vi "Actor Core.vi"(8 "error in":errorcluster, 11 "Example Actor in":refnum<class "Example Actor.lvclass">) -> (0 "error out":errorcluster, 3 "Actor out":refnum<class "Actor.lvclass">)   [LabVIEW 2021, in "Example Iterator NR Actor Explicit Iteration.lvlib" / "Example Actor.lvclass"]
doc: "(<B>Filename</B>: Actor Framework.lvlib:Actor.lvclass:Actor Core.vi)\n\nReceives messages to the actor, reacts to them, and initiates any error handling that may shut the actor down.\n\nDescendant classes may override this VI to append parallel tasks for the actor to complete while it handles messages. Overrides use the Call Parent Method node."
uses:
  Example Actor.lvclass
  C:/Program Files/National Instruments/LabVIEW 2021/vi.lib/ActorFramework/Actor/Actor.lvclass
  <vilib>/ActorFramework/Actor/Actor.lvclass
  Iterator Settings.ctl
  Abstract Iterator Actor/Active Stop Conditions.ctl
  Abstract Iterator Actor/Stop Reason.ctl
  Iterator NR Actor/Iterator NR Actor Folder/Iterator NR Actor.lvclass
  Example Actor.lvclass/Example Actor.ctl
  <vilib>/ActorFramework/Actor/Actor.lvclass/Actor.ctl
  <vilib>/ActorFramework/Message Enqueuer/Message Enqueuer.lvclass/Message Enqueuer.ctl
  Example Actor Messages/Iterate Reply Msg/Iteration Msg.lvclass
  C:/Program Files/National Instruments/LabVIEW 2021/vi.lib/ActorFramework/Message/Message.lvclass
  Abstract Iterator Actor/Iterator Settings.ctl
  <vilib>/ActorFramework/Message/Message.lvclass
  Iterator Actor/Iterator Actor Abstract Messages/Iterator Report Iterations End Msg/Iterator Report Iterations End Msg.lvclass
  Example Actor Messages/Pre Iterate Reply Msg/Pre Iteration Msg.lvclass
  Example Actor Messages/Post Iterate Reply Msg/Post Iteration Msg.lvclass
  Example Actor Messages/Update Error Msg/Update Error Msg.lvclass
  C:/Projects/Shared Libraries/Iterator Actor/Iterator Actor/Iterator Actor Abstract Messages/Iterator Report Iterations End Msg/Iterator Report Iterations End Msg.lvclass
  <vilib>/ActorFramework/Message Enqueuer/Init from Existing Queue.vi
  <vilib>/ActorFramework/Message Enqueuer/Enqueue.vi
  <vilib>/ActorFramework/Stop Msg/Stop Msg.lvclass
  <vilib>/ActorFramework/Message Priority Queue/Priority Enqueue.vi
  <vilib>/ActorFramework/Message Enqueuer/Message Enqueuer.lvclass
  Example Actor Messages/Write Ready for iterations Msg/Write Ready for iterations Msg.lvclass
  Iterator Actor/Iterator Actor Messages/Write Settings Msg/Write Settings Msg.lvclass
  Iterator Actor/Iterator Actor Messages/Start Iterations Msg/Start Iterations Msg.lvclass
  Iterator Actor/Iterator Actor Messages/Stop Iterations Msg/Stop Iterations Msg.lvclass
  Abstract Iterator Actor/Abstract Iterator Actor.lvclass
panel:
  out "Stop Reason":T1
  in  "Receive report":bool=TRUE
  in  "Do post-iterations":bool=TRUE
  in  "Do pre-iterations":bool=TRUE
  out "Iterator error":errorcluster
  in  "User Settings":T2={"Prepare timeout (ms)"=1000, "Iterate timeout (ms)"=1000, "Conclude timeout (ms)"=1000, "Iterate period (ms)"=1000, "Active Stop Conditions"={"Number of Iterations"=FALSE, "Time Elapsed"=FALSE, "Iteration Result"=FALSE}, "Iterations"=5, "Time before stop (ms)"=200}
  out "Post Iterate":bool
  out "Pre Iterate":bool
  in  "exit":bool
  out "Iterate":bool
  in  "stop iterations":bool
  in  "start iterations":bool
  in  "Ready for iterations":bool=TRUE
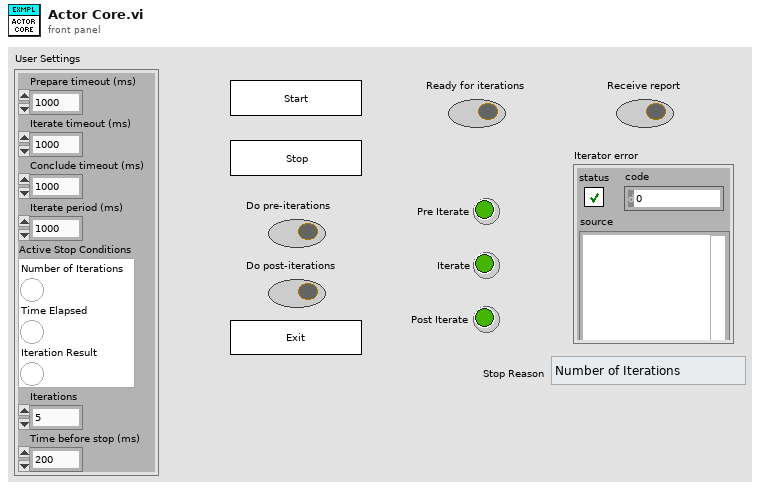
[diagram p1: front panel]
types:
  T1 = typedef "Iterator Actor.lvlib/Abstract Iterator Actor.lvclass/Stop Reason.ctl" = enum16{"Number of Iterations", "Time Elapsed", "Stopped Internally", "Stopped Externally"}
  T2 = typedef "Example Iterator NR Actor Explicit Iteration.lvlib/Example Actor.lvclass/Iterator Settings.ctl" = cluster{"Prepare timeout (ms)":i32, "Iterate timeout (ms)":i32, "Conclude timeout (ms)":i32, "Iterate period (ms)":i32, "Active Stop Conditions":T3, "Iterations":i32, "Time before stop (ms)":i32}
  T3 = typedef "Iterator Actor.lvlib/Abstract Iterator Actor.lvclass/Active Stop Conditions.ctl" = cluster{"Number of Iterations":bool, "Time Elapsed":bool, "Iteration Result":bool}
  T4 = typedef "Iterator Actor.lvlib/Abstract Iterator Actor.lvclass/Iterator Settings.ctl" = cluster{"Prepare timeout (ms)":i32, "Iterate timeout (ms)":i32, "Conclude timeout (ms)":i32, "Iterate period (ms)":i32, "Number of iterations":i32, "Time before stop (ms)":i32, "Active Stop Conditions":T3, "Prepare Msg":refnum<class "Message.lvclass">, "Iterate Msg":refnum<class "Message.lvclass">, "Conclude Msg":refnum<class "Message.lvclass">, "Iterations End Report":refnum<class "Iterator Report Iterations End Msg.lvclass">}
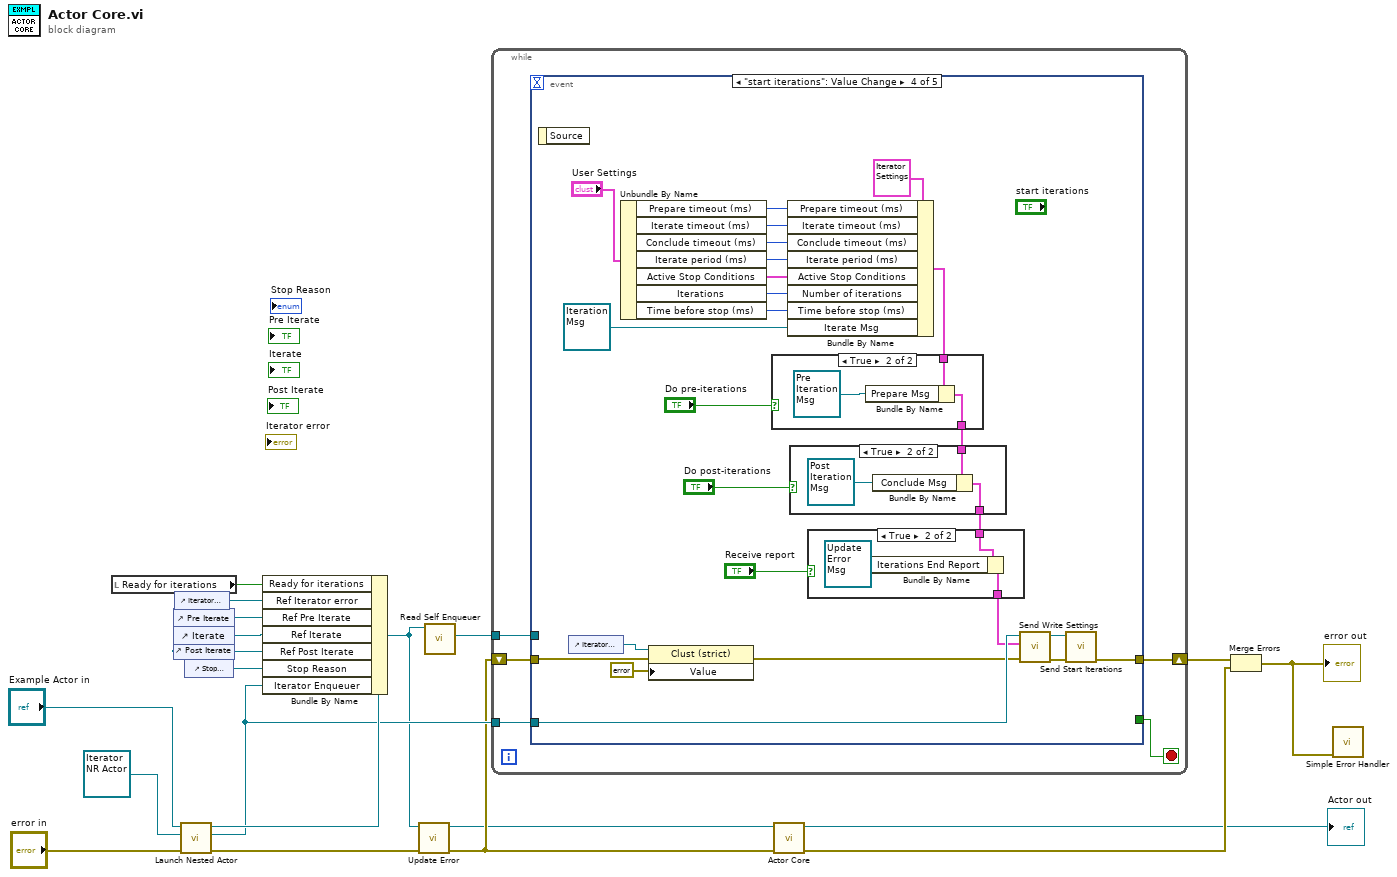
[diagram p0: block diagram]
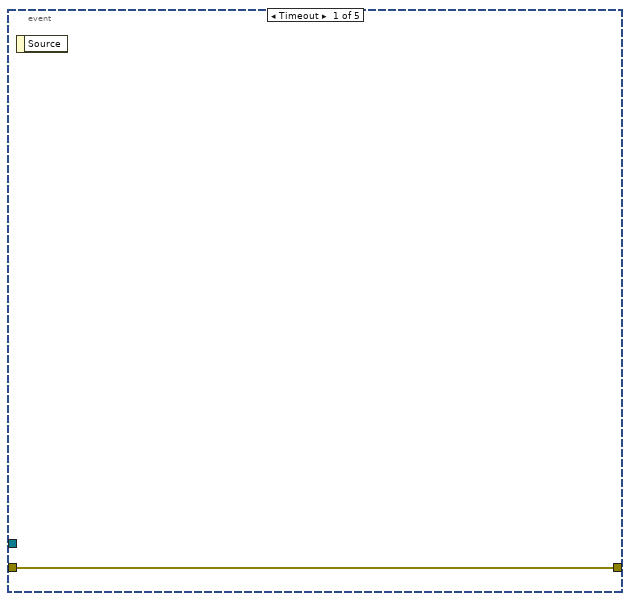
[diagram p2: hidden frame]
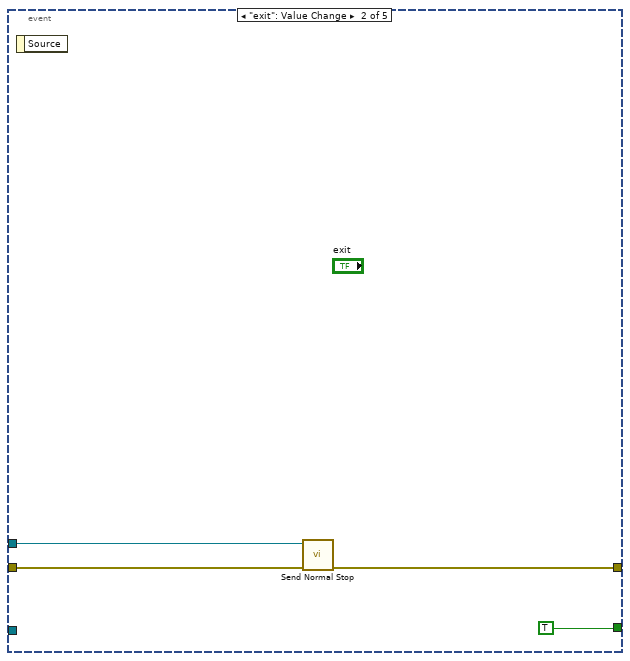
[diagram p3: hidden frame]
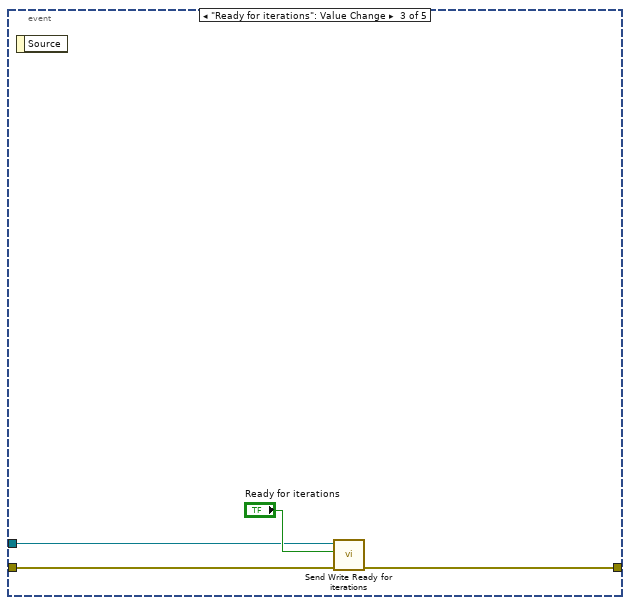
[diagram p4: hidden frame]
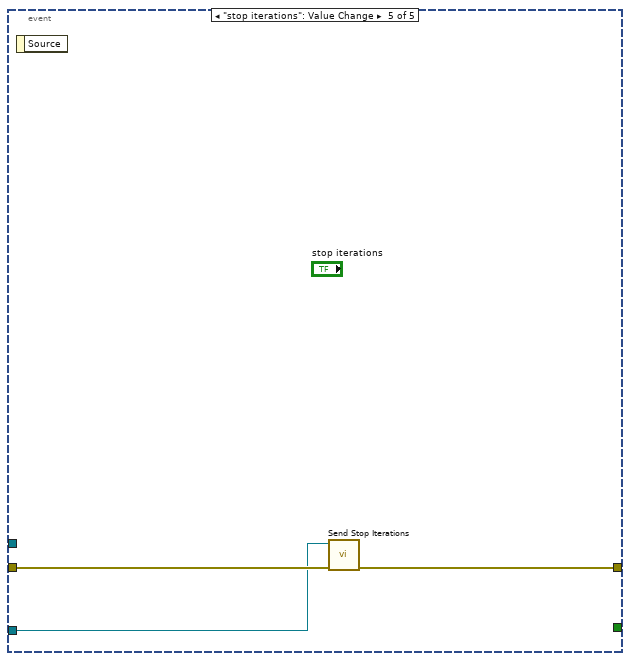
[diagram p8: hidden frame]
diagram:
  n1 = local read "Ready for iterations"() -> (w11:bool)
  n2 = control-ref of="Pre Iterate"() -> (w16:refnum<vi>)
  n3 = control-ref of="Iterate"() -> (w15:refnum<vi>)
  n4 = control-ref of="Post Iterate"() -> (w14:refnum<vi>)
  n5 = control-ref of="Iterator error"() -> (w9:refnum<vi>)
  n6 = call <vilib>:"Launch Nested Actor.vi"("error in (no error)"="error in", "Nested Actor"=refnum<class "Iterator NR Actor.lvclass"> refnum ("Iterator Actor 2.lvlib:Iterator Actor 2.lvclass"), "Caller Actor in"="Example Actor in") -> ("error out"=w8:errorcluster, "Nested Actor's Enqueuer"=w12:refnum<class "Message Enqueuer.lvclass">, "Caller Actor out"=w13:refnum<class "Example Actor.lvclass">)  [unwired: 6 in]
  n7 = control-ref of="Stop Reason"() -> (w4:refnum<vi>)
  n8 = Bundle By Name(cluster=w13, "Ready for iterations"=w11, "Ref Iterator error"=w9, "Ref Pre Iterate"=w16, "Ref Iterate"=w15, "Ref Post Iterate"=w14, "Stop Reason"=w4, "Iterator Enqueuer"=w12) -> (w6:refnum<class "Example Actor.lvclass">)
  n9 = call "Update Error.vi"("error in (no error)"=w8, "Example Actor in"=w6) -> ("error out"=w7:errorcluster, "Example Actor out"=w5:refnum<class "Example Actor.lvclass">)  [unwired: 8 in]
  n10 = call <vilib>:"Read Self Enqueuer.vi"("Actor"=w6) -> ("Self Enqueuer"=w20:refnum<class "Message Enqueuer.lvclass">)  [unwired: 10 in]
  n11 = while {
    tunnel: w20 -> [w25]
    shift-right: [w24] -> w19
    shift-left: w7 -> [w23]
    tunnel: w12 -> [w21]
    stop <- w22 stop-if-true
    n12 = event shown="[3] \"start iterations\": Value Change" {
      selector: _ -> [_ _ _ _ _]
      dyn-events: _ -> [_ _ _ _ _]
      timeout: _ -> [_ _ _ _ _]
      tunnel: w25 -> [_ w30 w31 _ _]
      tunnel: [w26 w29 w32 w44 w73] -> w24
      tunnel: w23 -> [w26 w28 w34 w47 w74]
      tunnel: [_ TRUE _ _ _] -> w22
      tunnel: w21 -> [_ _ _ w58 w72]
      event Timeout {
        n13 = event-data() -> ()  [unwired: 1 in, 1 out]
      }
      event "exit": Value Change {
        n14 = event-data() -> ()  [unwired: 1 in, 1 out]
        n15 = call <vilib>:"Send Normal Stop.vi"("error in (no error)"=w28, "Message Enqueuer"=w30) -> ("error out"=w29:errorcluster)  [unwired: 9 in]
      }
      event "Ready for iterations": Value Change {
        n16 = event-data() -> ()  [unwired: 1 in, 1 out]
        n17 = call "Send Write Ready for iterations.vi"("error in (no error)"=w34, "Ready for iterations"="Ready for iterations", "Message Enqueuer in"=w31) -> ("error out"=w32:errorcluster)  [unwired: 7 in, 1 out]
      }
      event "start iterations": Value Change {
        n18 = event-data() -> ()  [unwired: 1 in, 1 out]
        n19 = control-ref of="Iterator error"() -> (w46:refnum<vi>)
        n20 = Unbundle By Name("User Settings") -> ("Prepare timeout (ms)"=w51:i32, "Iterate timeout (ms)"=w52:i32, "Conclude timeout (ms)"=w53:i32, "Iterate period (ms)"=w54:i32, "Active Stop Conditions"=w48:T3, "Iterations"=w49:i32, "Time before stop (ms)"=w50:i32)
        n21 = property class="Clust (strict)"(reference=w46, error in=w47, "Value"=errorcluster {"status"=FALSE, "code"=0, "source"=""}) -> (error out=w42:errorcluster)  [unwired: 1 out]
        n22 = Bundle By Name(cluster=T4 {"Prepare timeout (ms)"=0, "Iterate timeout (ms)"=0, "Conclude timeout (ms)"=0, "Iterate period (ms)"=0, "Number of iterations"=0, "Time before stop (ms)"=0, "Active Stop Conditions"={"Number of Iterations"=FALSE, "Time Elapsed"=FALSE, "Iteration Result"=FALSE}, "Prepare Msg"=refnum, "Iterate Msg"=refnum, "Conclude Msg"=refnum, "Iterations End Report"=refnum} ("Iterator Settings"), "Prepare timeout (ms)"=w51, "Iterate timeout (ms)"=w52, "Conclude timeout (ms)"=w53, "Iterate period (ms)"=w54, "Active Stop Conditions"=w48, "Number of iterations"=w49, "Time before stop (ms)"=w50, "Iterate Msg"=refnum<class "Iteration Msg.lvclass"> refnum ("Example Actor.lvlib:Iterate Reply Msg.lvclass")) -> (w39:T4)
        n23 = case shown="True" "Do pre-iterations" {
          tunnel: w39 -> [w68 w71]
          tunnel: [w68 w69] -> w38
          frame False {
          }
          frame True {
            n24 = Bundle By Name(cluster=w71, "Prepare Msg"=refnum<class "Pre Iteration Msg.lvclass"> refnum ("Example Actor.lvlib:Pre Iterate Reply Msg.lvclass")) -> (w69:T4)
          }
        }
        n25 = case shown="True" "Do post-iterations" {
          tunnel: w38 -> [w64 w67]
          tunnel: [w64 w65] -> w36
          frame False {
          }
          frame True {
            n26 = Bundle By Name(cluster=w67, "Conclude Msg"=refnum<class "Post Iteration Msg.lvclass"> refnum ("Example Actor.lvlib:Post Iterate Reply Msg.lvclass")) -> (w65:T4)
          }
        }
        n27 = case shown="True" "Receive report" {
          tunnel: [w60 w63] -> w35
          tunnel: w36 -> [w60 w62]
          frame False {
          }
          frame True {
            n28 = Bundle By Name(cluster=w62, "Iterations End Report"=refnum<class "Update Error Msg.lvclass"> refnum ("Example Actor.lvlib:Update Error Msg.lvclass")) -> (w63:T4)
          }
        }
        n29 = call "Send Write Settings.vi"("error in (no error)"=w42, "Settings"=w35, "Message Enqueuer in"=w58) -> ("error out"=w59:errorcluster, "Message Enqueuer out"=w43:refnum<class "Message Enqueuer.lvclass">)  [unwired: 7 in]
        n30 = call "Send Start Iterations.vi"("error in (no error)"=w59, "Message Enqueuer in"=w43) -> ("error out"=w44:errorcluster)  [unwired: 8 in, 1 out]
      }
      event "stop iterations": Value Change {
        n31 = event-data() -> ()  [unwired: 1 in, 1 out]
        n32 = call "Send Stop Iterations.vi"("error in (no error)"=w74, "Message Enqueuer in"=w72) -> ("error out"=w73:errorcluster)  [unwired: 8 in, 1 out]
      }
    }
  }
  n33 = call-parent "Actor Core.vi"("error in"=w7, "Actor in"=w5) -> ("error out"=w18:errorcluster, "Actor out"=→"Actor out":refnum<class "Actor.lvclass">)  [unwired: 8 in]
  n34 = Merge Errors(w19, w18) -> (w10:errorcluster)
  "error out" <- w10
  n35 = call <vilib>:"Simple Error Handler.vi"("error in (no error)"=w10) -> ()  [unwired: 4 in, 5 out]
